vi "AlliGator Save ROI(s).vi"(7 "Current Dataset Name":string="Source Image", 8 "Error In":errorcluster, 9 "ROI Descriptor":T1 {"Contours"."Type" items=["No Selection", "Point", "Line", "Rectangle", "Oval", "Polygon", "Freehand Region", "Annulus", "Unused2", "Unused3", "Broken Line", "Freehand Line", "Rotated Rectangle"]}, 10 "All ROIs?":bool=TRUE, 11 "Image Label":string="Source Image") -> (0 "Error Out":errorcluster, 2 "Message":string)   [LabVIEW 2021, in "AlliGator ROIs.lvlib"]
doc: "Saves one or more ROIs."
uses:
  AlliGator ROIs.lvlib
  AlliGator ROI Manager Actions.ctl
  Image/Named ROI Description.ctl
  Image/Image Control Multiple ROIs Description v2.ctl
  Globals, Variables, Constants/AlliGator Variables List.ctl
  AlliGator Phasor Plot Image ROI Storage [SGL] v3.vi
  AlliGator Source Image ROI Storage [SGL] v3.vi
  Image/Image.lvlib
  Globals, Variables, Constants/AlliGator Globals, Variables & Constants.lvlib
panel:
  # "see the AlliGator License on the block diagram (Ctrl+E or Window:Show Block Diagram)"
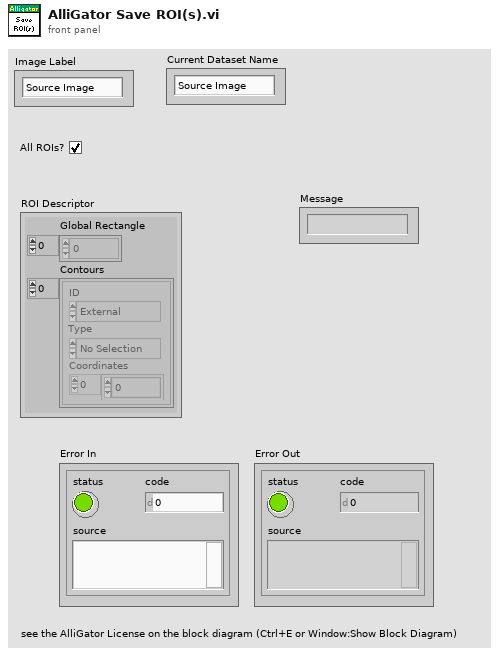
[diagram p1: front panel]
types:
  T1 = typedef "ROI Descriptor" = cluster{"Global Rectangle":i32[], "Contours":cluster{"ID":enum32{"External", "Internal"}, "Type":u32, "Coordinates":i32[]}[]}
  T2 = typedef "AlliGator ROIs.lvlib/AlliGator ROI Manager Actions.ctl" = enum16{"Undefined", "Delete Current ROI", "Delete All Unselected ROIs", "Delete Multiple ROIs", "Delete All ROIs", "Swap ROIs", "Insert ROI", "Update Current ROI Descriptor", "Rename Current ROI", "Store New ROI", "Store Multiple ROIs", "Select Next ROI", "Select Previous ROI", "Find Selected ROI", "Show All ROIs", "Update ROI Manager Window", "Merge All ROIs", "Unmerge ROI", "Set Selected ROI by ID"}
  T3 = typedef "Image.lvlib/Named ROI Description.ctl" = cluster{"ROI Descriptor":T1, "ROI Name":string, "Overlay Color":u32}
  T4 = typedef "Image.lvlib/Image Control Multiple ROIs Description v2.ctl" = cluster{"Image Control Label":string, "Named ROI Descriptions":T3[]}
  T5 = typedef "AlliGator Globals, Variables & Constants.lvlib/AlliGator Variables List.ctl" = enum16{"---- GUI ----", "GUI:Initialization Status", "GUI:State Indicators Refnum", "GUI:Original AlliGator Menu Items", "GUI:Current Action Loop State", "GUI:Script in progress", "GUI:Playback", "GUI:Loop Playback", "GUI:Search ROI Used", "GUI:Search ROI", "Decay Graph Max Legend Size", "Intensity Graph Max Legend Size", "Decay Statistics Graph Max Legend Size", "Phasor Graph Max Legend Size", "Phasor Ratio Graph Max Legend Size", "Lifetime Graph Max Legend Size", "---- Files ----", "Files:Export Dataset Frames as Individual Files", "Files:Show Batch Export Help Balloons", "Files:Frames in Dataset", "Files:ptu File Frame Start Indices", "Files:Current Frame in Dataset", "Files:Current Frame Timestamp", "Files:Dataset Loaded", "Files:Dataset Metadata", "Files:Dataset Channel", "Files:Dataset Data Description", "Files:Background Dataset Metadata", "Files:Background Dataset Channel", "Files:Background Dataset Data Description", "Files:Background File Subtraction", "Files:Background File Path", "Files:Background File Pile-up Correction", "Files:Background File Pixel Well Capacity", "Files:Background File Scaling Factor", "Files:Current Dataset Load Settings", "Files:Dataset Path", "Files:ICCD-specific Information", "Files:Macrotime Gate Separation", "------ Python Plugins ------", "Python Plugins:Information", "Python Plugins:Python Session", "Python Plugins:Valid Python Session?", "---- Source Image ----", "Source Image:ROIs", "Source Image:Current ROI", "Source Image:ROI Event Refnum", "X_Source Image Display Range", "X_Source Image Palette Information", "X_Type of Displayed Image", "X_Time Gate Slider", "Source Image:Palette List", "Source Image:Scale", "Source Image:ROI Overlay Color", "Source Image:Overlay to Erase", "Source Image:Is Displayed Image Accumulated", "Source Image:White Light Image Modified", "Source Image:Mask Image Modified", "---- Image Profile Window ----", "Image Profile:Window Event Refnum", "Image Profile:IntensityType", "Image Profile:Intensity Average Type", "Image Profile:Intensity-weighted SDV", "Image Profile:Box Profile Type", "Image Profile:Window Open", "Image Profile:Plotted Fit Parameter", "------ Phasor Graph -------", "Phasor Graph:Show Line", "---- Phasor Plot ---", "Phasor Plot:Parameters Changed", "Phasor Plot:FLI Dataset Modified since last Calculation", "Phasor Harmonics Data", "Selected Phasor Harmonics", "Phasor Harmonic Manager Event Refnum", "Phasor Plot:ROIs", "Phasor Plot:Current ROI", "Phasor Plot:ROI Event Refnum", "Phasor Plot:Image Reference Points", "Phasor Plot:Computed", "Phasor Plot:Palette Information", "Phasor Plot:Palette List", "Phasor Plot:Phasor Ratio Palette Information", "Phasor Plot:Phasor Ratio Palette List", "Phasor Plot:Image Scale", "Phasor Plot:Image Overlay to Erase", "Phasor Plot:Image Elements to Update", "Phasor Plot:Current Calculation Parameters", "Phasor Plot:Current Calibration Options", "Phasor Plot:Reset Cumulated Phasor Plot", "Phasor Plot:Reference 1", "Phasor Plot:Lifetime Reference 1", "Phasor Plot:Reference 1 Frequency", "Phasor Plot:Reference 2", "Phasor Plot:Lifetime Reference 2", "Phasor Plot:Reference 2 Frequency", "---- Decay Analysis ----", "Number of Selected Decays to Fit", "LS Fit Results", "LAR Fit Results", "BS Fit Results", "Last Decay Max - Min", "Best Fit Parameters", "Best Fit Parameter Names", "Actual Size X", "Actual Size Y", "Binning X", "Binning Y", "Actual # Gates", "Dataset Number", "Gates to...", "Gates Skipped", "Gates to keep", "Gate Step", "Gate Separation", "Reversed Gates", "Pile-up Correction", "Pixel Well Capacity", "Background Subtracted", "Background Subtraction Method", "Background Definition Range", "Background File (deprecated)", "Number of Dataset Accumulated", "Array of Accumulated Dataset Paths", "Do Averaged Datasets", "Destination File Path", "Process Plot Target", "Use 1/D as Phasor Frequency", "---- Decay Fit Parameter Map -----", "Decay Fit Parameter Map:Palette Information", "Decay Fit Parameter Map:Palette List", "---- Parameter Map ----", "Parameter Map:Palette Information", "Parameter Map:Palette List", "------- Local Decay Window ---------", "Local Decay Graph Window:Event Refnum", "Local Decay Graph Window:Use normalized IRF for convolution", "----- Miscellaneous ----", "Misc:Skippable Dialog Windows Status"}
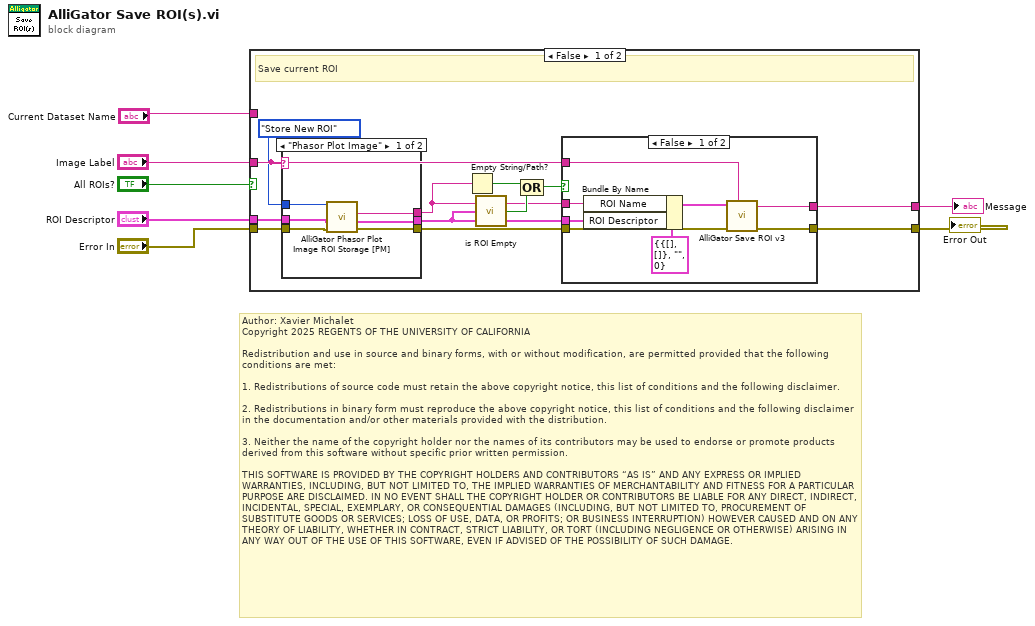
[diagram p0: block diagram]
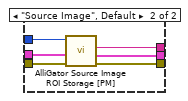
[diagram p2: hidden frame]
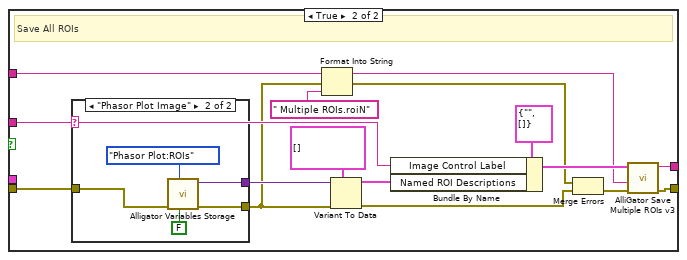
[diagram p4: hidden frame]
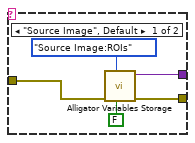
[diagram p5: hidden frame]
diagram:
  # "Author: Xavier Michalet\nCopyright 2025 REGENTS OF THE UNIVERSITY OF CALIFORNIA\n\nRedistribution and use in source and binary forms, with or without modification, are permitted provided that the following conditions are met:\n\n1. Redistributions of source code must retain the above copyright notice, this list of conditions and the following disclaimer.\n\n2. Redistributions in binary form must reproduce the above copyright notice, this list of conditions and the following disclaimer in the documentation and/or other materials provided with the distribution.\n\n3. Neither the name of the copyright holder nor the names of its contributors may be used to endorse or promote products derived from this software without specific prior written permission.\n\nTHIS SOFTWARE IS PROVIDED BY THE COPYRIGHT HOLDERS AND CONTRIBUTORS “AS IS” AND ANY EXPRESS OR IMPLIED WARRANTIES, INCLUDING, BUT NOT LIMITED TO, THE IMPLIED WARRANTIES OF MERCHANTABILITY AND FITNESS FOR A PARTICULAR PURPOSE ARE DISCLAIMED. IN NO EVENT SHALL THE COPYRIGHT HOLDER OR CONTRIBUTORS BE LIABLE FOR ANY DIRECT, INDIRECT, INCIDENTAL, SPECIAL, EXEMPLARY, OR CONSEQUENTIAL DAMAGES (INCLUDING, BUT NOT LIMITED TO, PROCUREMENT OF SUBSTITUTE GOODS OR SERVICES; LOSS OF USE, DATA, OR PROFITS; OR BUSINESS INTERRUPTION) HOWEVER CAUSED AND ON ANY THEORY OF LIABILITY, WHETHER IN CONTRACT, STRICT LIABILITY, OR TORT (INCLUDING NEGLIGENCE OR OTHERWISE) ARISING IN ANY WAY OUT OF THE USE OF THIS SOFTWARE, EVEN IF ADVISED OF THE POSSIBILITY OF SUCH DAMAGE."
  n1 = case shown="False" "All ROIs?" {
    tunnel: "Error In" -> [w10 w53]
    tunnel: [w19 w55] -> w2
    tunnel: [w18 w56] -> w3
    tunnel: "Image Label" -> [w9 w47]
    tunnel: "ROI Descriptor" -> [w14 _]
    tunnel: "Current Dataset Name" -> [_ w45]
    frame False {
      # "Save current ROI"
      n2 = case shown="\"Phasor Plot Image\"" w9 {
        tunnel: w14 -> [w25 w31]
        tunnel: [w21 w30] -> w13
        tunnel: [w22 w29] -> w12
        tunnel: [w23 w28] -> w11
        tunnel: w10 -> [w24 w27]
        tunnel: AlliGator_ROI_Manager_Actions."Store New ROI" ("Action") -> [w20 w26]
        frame "Phasor Plot Image" {
          n3 = call-poly "AlliGator Phasor Plot Image ROI Storage [PM].vi"("Error In"=w24, "Current ROI Descriptor"=w25, "Action"=w20) -> ("Error Out"=w21:errorcluster, "Current ROI Descriptor"=w22:T1, "Current ROI Name"=w23:string)  [unwired: 3 in, 3 out]
        }
        frame "Source Image", Default {
          n4 = call-poly "AlliGator Source Image ROI Storage [PM].vi"("Error In"=w27, "Current ROI Descriptor"=w31, "Action"=w26) -> ("Error Out"=w30:errorcluster, "Current ROI Descriptor"=w29:T1, "Current ROI Name"=w28:string)  [unwired: 2 in, 4 out]
        }
      }
      n5 = Empty String/Path?(string/path=w11) -> (empty?=w17:bool)
      n6 = call "is ROI Empty.vi"("Current ROI Descriptor"=w12) -> ("Empty ROI?"=w16:bool)  [unwired: 8 in]
      n7 = Compound Arithmetic op=OR(w17, w16) -> (w15:bool)
      n8 = case shown="False" w15 {
        tunnel: [w37 w40] -> w19
        tunnel: [w36 _] -> w18
        tunnel: w9 -> [w35 _]
        tunnel: w13 -> [w34 w40]
        tunnel: w12 -> [w33 _]
        tunnel: w11 -> [w32 _]
        frame False {
          n9 = Bundle By Name(cluster=T3 {"ROI Descriptor"={"Global Rectangle"=[], "Contours"=[]}, "ROI Name"="", "Overlay Color"=0} ("ROI Description"), "ROI Name"=w32, "ROI Descriptor"=w33) -> (w38:T3)
          n10 = call "AlliGator Save ROI v3.vi"("Image Label"=w35, "Error In"=w34, "ROI Description"=w38) -> ("Error Out"=w37:errorcluster, "Notebook Message"=w36:string)  [unwired: 7 in]
        }
        frame True {
        }
      }
    }
    frame True {
      # "Save All ROIs"
      n11 = case shown="\"Phasor Plot Image\"" w47 {
        tunnel: [w59 w64] -> w54
        tunnel: [w58 w63] -> w46
        tunnel: w53 -> [w57 w62]
        frame "Source Image", Default {
          n12 = call "Alligator Variables Storage.vi"("Get(F)/Set"=FALSE, "AlliGator Variable"=AlliGator_Variables_List."Source Image:ROIs" ("Alligator Variable"), "Error In"=w57) -> ("Error Out"=w58:errorcluster, "Data out"=w59:variant)  [unwired: 6 in, 1 out]
        }
        frame "Phasor Plot Image" {
          n13 = call "Alligator Variables Storage.vi"("Get(F)/Set"=FALSE, "AlliGator Variable"=AlliGator_Variables_List."Phasor Plot:ROIs" ("Alligator Variable"), "Error In"=w62) -> ("Error Out"=w63:errorcluster, "Data out"=w64:variant)  [unwired: 6 in, 1 out]
        }
      }
      n14 = Format Into String(initial string=w45, error in=w46, " Multiple ROIs.roiN" ("input 1")) -> (resulting string=w43:string, error out=w41:errorcluster)  [unwired: 1 in]
      n15 = Variant To Data(error in=w46, type=T3[] [] ("ROIs"), Variant=w54) -> (data=w50:T3[], error out=w52:errorcluster)
      n16 = Bundle By Name(cluster=T4 {"Image Control Label"="", "Named ROI Descriptions"=[]} ("Image Control ROI Descriptions"), "Image Control Label"=w47, "Named ROI Descriptions"=w50) -> (w48:T4)
      n17 = Merge Errors(w41, w52) -> (w42:errorcluster)
      n18 = call "AlliGator Save Multiple ROIs v3.vi"("Error In"=w42, "Default File Name"=w43, "ROI Description"=w48) -> ("Error Out"=w55:errorcluster, "Notebook Message"=w56:string)  [unwired: 7 in]
    }
  }
  "Error Out" <- w2
  "Message" <- w3
